vi "report results.vi"(8 "error in":errorcluster, 10 "result":refnum<class "result.lvclass">, 11 "queue reporter in":refnum<class "queue reporter.lvclass">) -> (0 "error out":errorcluster, 3 "queue reporter out":refnum<class "queue reporter.lvclass">)   [LabVIEW 2013, in "queue reporter.lvclass"]
uses:
  queue reporter.lvclass
  result/result.lvclass
  queue reporter.lvclass/queue reporter.ctl
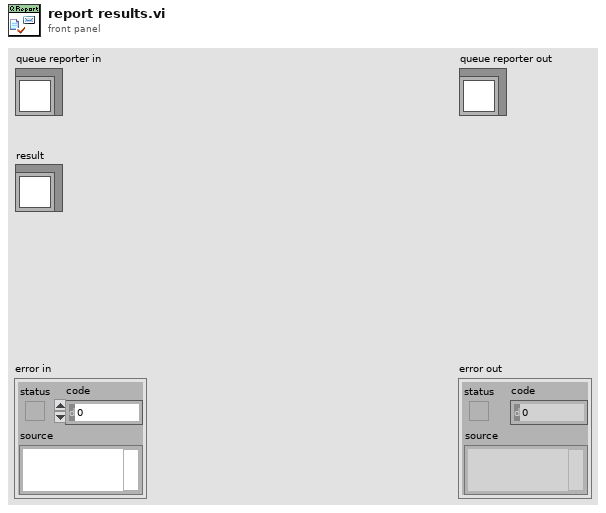
[diagram p1: front panel]
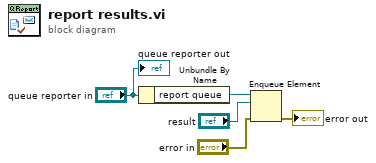
[diagram p0: block diagram]
diagram:
  n1 = Unbundle By Name("queue reporter in") -> ("report queue"=w2:refnum<queue>)
  n2 = Enqueue Element(queue=w2, element="result", error in (no error)="error in") -> (error out=→"error out":errorcluster)  [unwired: 1 in, 2 out]
  "queue reporter out" <- "queue reporter in"
